vi "VI.vi"(1 "In":variant, 2 "Names":string[][](array[string]), 3 "Path":path, 4 "Mode":u32(ring) items=["Open", "Close", "Begin", "End", "Get", "Set"]) -> (0 "Out":variant)   [LabVIEW 2014]
panel:
  out "Units":string[](array[string])
  out "Ctrls":refnum<vi>[](array[refnum])
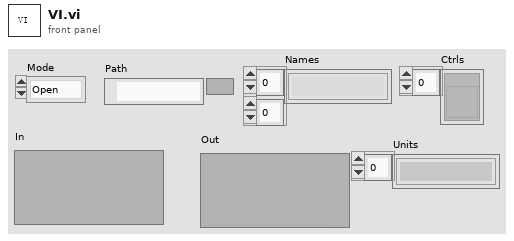
[diagram p1: front panel]
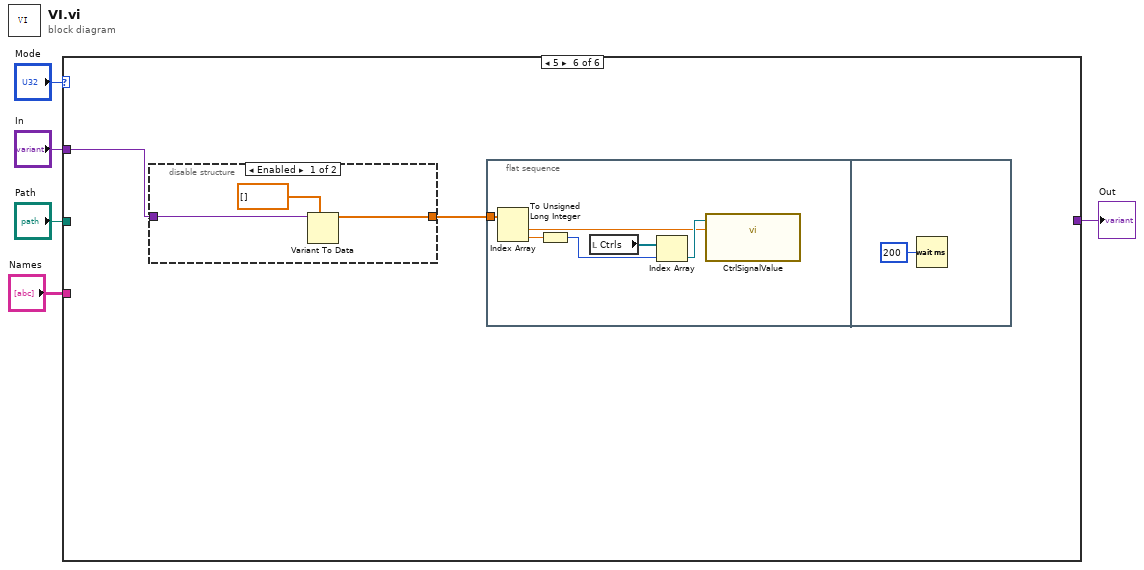
[diagram p0: block diagram]
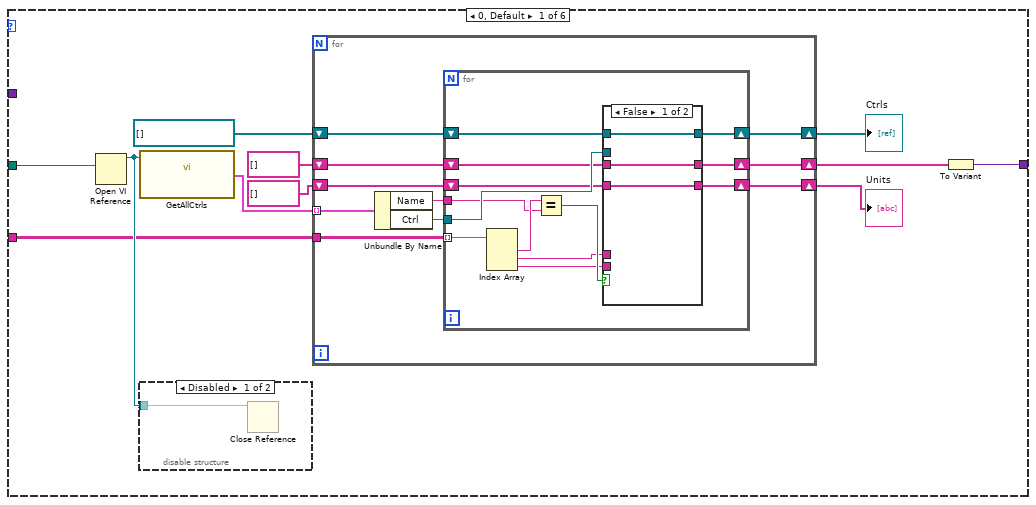
[diagram p2: hidden frame]
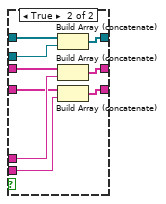
[diagram p4: hidden frame]
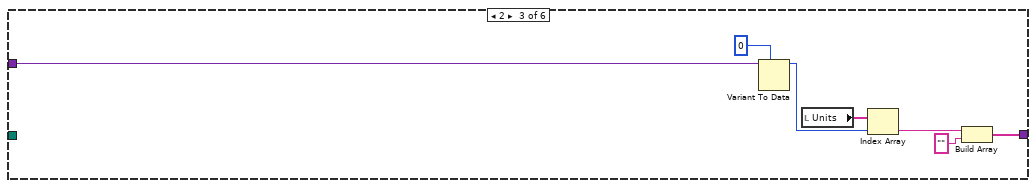
[diagram p6: hidden frame]
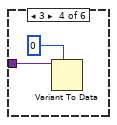
[diagram p7: hidden frame]
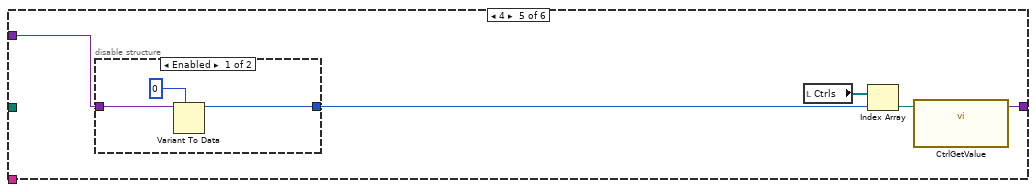
[diagram p8: hidden frame]
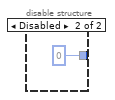
[diagram p9: hidden frame]
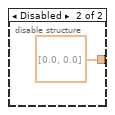
[diagram p10: hidden frame]
diagram:
  n1 = case shown="5" "Mode" {
    tunnel: "In" -> [_ _ w59 w60 w66 w72]
    tunnel: [w16 _ w56 _ w63 _] -> w4
    tunnel: "Path" -> [w15 _ _ _ _ _]
    tunnel: "Names" -> [w11 _ _ _ _ _]
    frame 0, Default {
      n2 = Open VI Reference(vi path=w15) -> (vi reference=w12:refnum<vi>)  [unwired: 5 in, 1 out]
      n3 = call "GetAllCtrls.vi"("VI"=w12) -> ("Ctrls"=w9:cluster{"Name":string, "Ctrl":refnum<vi>}[])  [unwired: 1 in]
      n4 = disable-structure shown="Disabled" {
        disable-tunnel: w12 -> [w17 _]
        frame Disabled {
          n5 = Close Reference(reference=w17) -> ()  [unwired: 1 in, 1 out]
        }
        frame Enabled {
        }
      }
      n6 = for {
        tunnel: w9 -> [w27] mode=indexing
        shift-right: [w23] -> w13
        shift-left: refnum<vi>[] [] ("Ctrls") -> [w22]
        tunnel: w11 -> [w26]
        shift-right: [w20] -> w14
        shift-left: string[] [] -> [w21]
        shift-right: [w18] -> w10
        shift-left: string[] [] -> [w19]
        n7 = Unbundle By Name(w27) -> ("Name"=w25:string, "Ctrl"=w24:refnum<vi>)
        n8 = for {
          tunnel: w26 -> [w40] mode=indexing
          tunnel: w25 -> [w32]
          tunnel: w24 -> [w37]
          shift-right: [w36] -> w23
          shift-left: w22 -> [w35]
          shift-right: [w33] -> w20
          shift-left: w21 -> [w34]
          shift-right: [w28] -> w18
          shift-left: w19 -> [w29]
          n9 = Index Array(array=w40) -> (element #1=w39:string, element #2=w31:string, element #3=w30:string)  [unwired: 3 in]
          n10 = Equal?(x=w39, y=w32) -> (x = y?=w38:bool)
          n11 = case shown="False" w38 {
            tunnel: w37 -> [_ w52]
            tunnel: w35 -> [w43 w51]
            tunnel: [w43 w50] -> w36
            tunnel: w34 -> [w42 w48]
            tunnel: [w42 w49] -> w33
            tunnel: w31 -> [_ w47]
            tunnel: w30 -> [_ w46]
            tunnel: w29 -> [w41 w45]
            tunnel: [w41 w44] -> w28
            frame False {
            }
            frame True {
              n12 = Build Array (concatenate)(w51, w52) -> (w50:refnum<vi>[])
              n13 = Build Array (concatenate)(w48, w47) -> (w49:string[])
              n14 = Build Array (concatenate)(w45, w46) -> (w44:string[])
            }
          }
        }
      }
      "Ctrls" <- w13
      "Units" <- w10
      n15 = To Variant(anything=w14) -> (Variant=w16:variant)
    }
    frame 1 {
    }
    frame 2 {
      n16 = Variant To Data(type=0, Variant=w59) -> (data=w54:i32)  [unwired: 1 in, 1 out]
      n17 = local read "Units"() -> (w55:string[])
      n18 = Index Array(array=w55, index=w54) -> (element=w53:string)
      n19 = Build Array(w53, "") -> (w56:string[])
    }
    frame 3 {
      n20 = Variant To Data(type=0, Variant=w60) -> ()  [unwired: 1 in, 2 out]
    }
    frame 4 {
      n21 = disable-structure shown="Enabled" {
        disable-tunnel: w66 -> [w69 _]
        disable-tunnel: [w67 0 ("index")] -> w62
        frame Enabled {
          n22 = Variant To Data(type=u32 0, Variant=w69) -> (data=w67:u32)  [unwired: 1 in, 1 out]
        }
        frame Disabled {
        }
      }
      n23 = local read "Ctrls"() -> (w65:refnum<vi>[])
      n24 = Index Array(array=w65, index=w62) -> (element=w64:refnum<vi>)
      n25 = call "CtrlGetValue.vi"("reference"=w64) -> ("variant"=w63:variant)  [unwired: 1 in, 3 out]
    }
    frame 5 {
      n26 = disable-structure shown="Enabled" {
        disable-tunnel: w72 -> [w82 _]
        disable-tunnel: [w80 dbl[] [0.0, 0.0] ("appended array")] -> w71
        frame Enabled {
          n27 = Variant To Data(type=dbl[] [] ("appended array"), Variant=w82) -> (data=w80:dbl[])  [unwired: 1 in, 1 out]
        }
        frame Disabled {
        }
      }
      n28 = flat-sequence {
        tunnel: w71 -> [w78]
        frame #0 {
          n29 = Index Array(array=w78) -> (element #1=w73:dbl, element #2=w77:dbl)  [unwired: 2 in]
          n30 = To Unsigned Long Integer(number=w77) -> (unsigned 32bit integer=w76:u32)
          n31 = local read "Ctrls"() -> (w75:refnum<vi>[])
          n32 = Index Array(array=w75, index=w76) -> (element=w74:refnum<vi>)
          n33 = call "CtrlSignalValue.vi"("variant"=w73, "reference"=w74) -> ()  [unwired: 2 in, 1 out]
        }
        frame #1 {
          n34 = Wait (ms)(milliseconds to wait=u32 200) -> ()  [unwired: 1 out]
        }
      }
    }
  }
  "Out" <- w4
